vi "Scan Setup.vi"(8 "error in (no error)":errorcluster, 11 "Translation Stage in":refnum<class "Translation Stage.lvclass">) -> (0 "error out":errorcluster, 3 "Translation Stage out":refnum<class "Translation Stage.lvclass">)   [LabVIEW 2017, in "Translation Stage.lvclass"]
uses:
  Translation Stage.lvclass
  Translation Stage.lvclass/Translation Stage.ctl
  Global/GPIB Numbers.vi
  Scanner/Scanner.lvclass
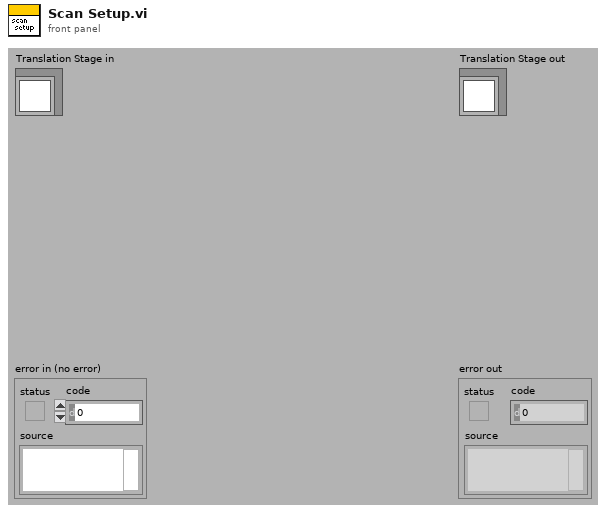
[diagram p1: front panel]
types:
  T1 = typedef "GPIB Type Def.ctl" = cluster{"Name":string, "bus":dbl, "GPIB":dbl, "GPIB as string":string, "byte":i32, "VISA Resource Name":refnum<visa-resource-name>}
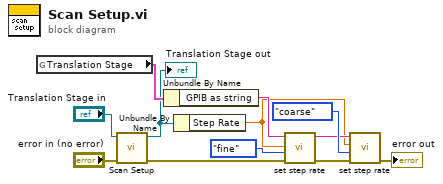
[diagram p0: block diagram]
diagram:
  n1 = global read "GPIB Numbers.vi" "Translation Stage"() -> (w8:T1)
  n2 = call-parent "Scan Setup.vi"("error in (no error)"="error in (no error)", "Scanner in"="Translation Stage in") -> ("error out"=w10:errorcluster, "Scanner out"=w6:refnum<class "Translation Stage.lvclass">)  [unwired: 8 out]
  "Translation Stage out" <- w6
  n3 = Unbundle By Name(w8) -> ("GPIB as string"=w7:string)
  n4 = Unbundle By Name(w6) -> ("Step Rate"=w1:dbl)
  n5 = call "set step rate.vi"("error in"=w10, "axis (def: fine)"=enum16{"fine", "coarse"}."fine", "step rate"=w1, "GPIB # (in): def. 6"=w7) -> ("error out"=w5:errorcluster, "GPIB # (out)"=w2:string)  [unwired: 6 out]
  n6 = call "set step rate.vi"("error in"=w5, "axis (def: fine)"=enum16{"fine", "coarse"}."coarse", "step rate"=w1, "GPIB # (in): def. 6"=w2) -> ("error out"=→"error out":errorcluster)  [unwired: 7 out]
